vi "采水流程.vi"(11 "参数设置":cluster{"排空时间":dbl, "润洗时间":dbl, "进样超时时间":dbl}={"排空时间"=120.0, "润洗时间"=120.0, "进样超时时间"=300.0}) -> ()   [LabVIEW 2016, in "环境动力单元.lvlib"]
panel:
  in  "排空初始化":bool
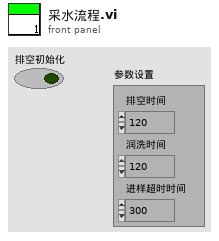
[diagram p1: front panel]
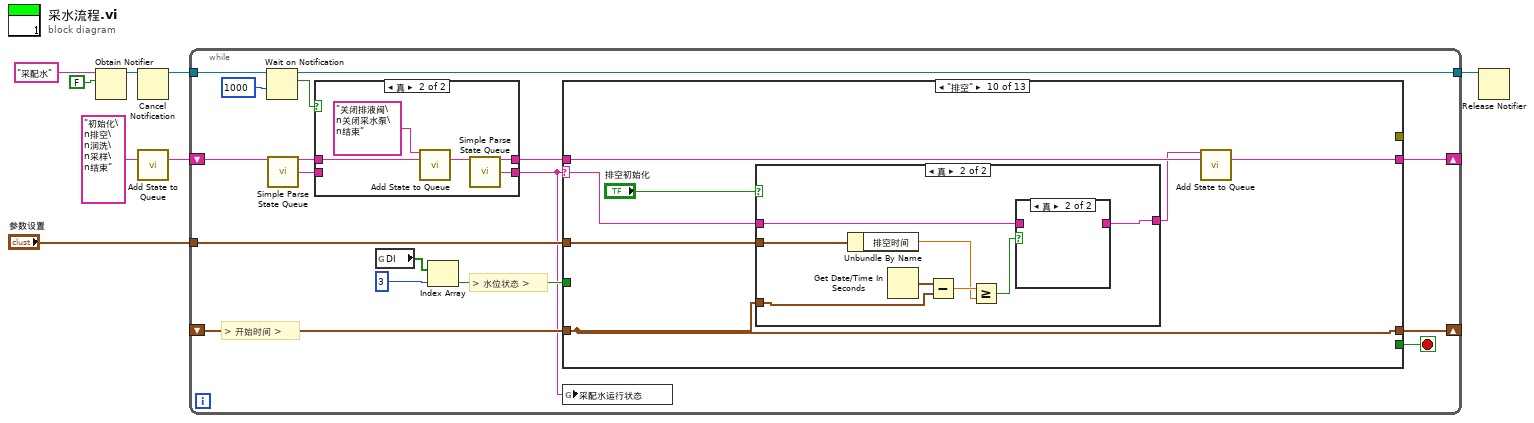
[diagram p0: block diagram]
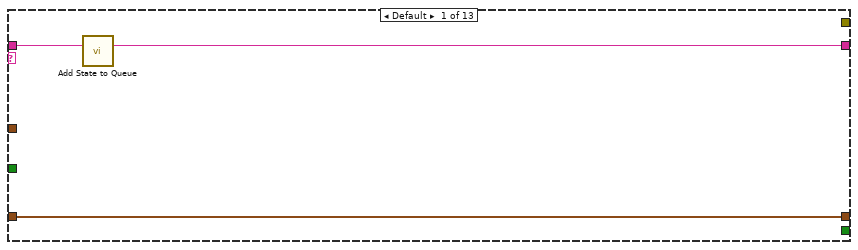
[diagram p3: hidden frame]
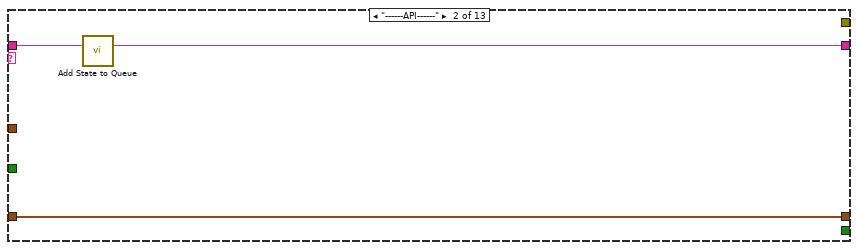
[diagram p4: hidden frame]
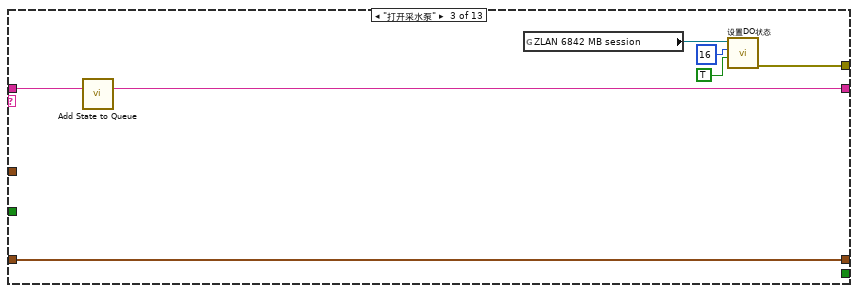
[diagram p5: hidden frame]
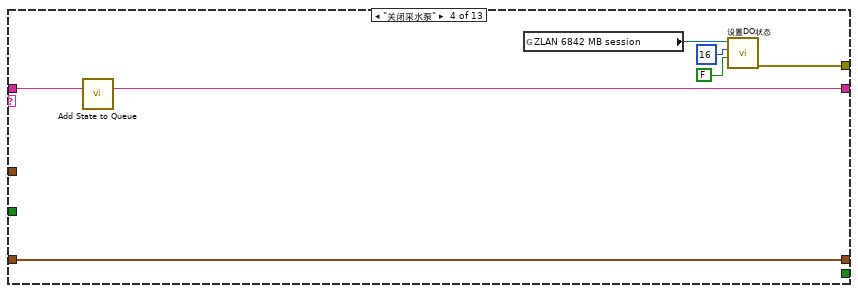
[diagram p6: hidden frame]
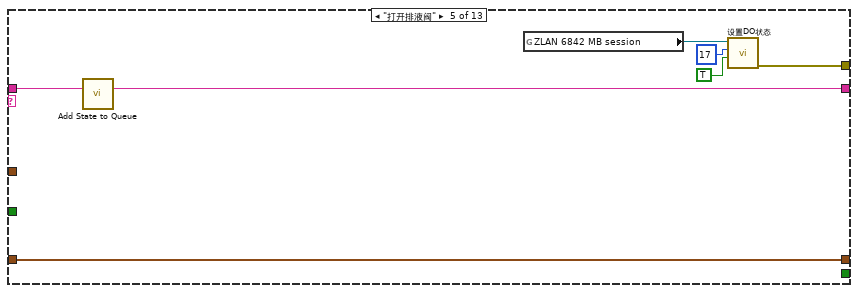
[diagram p7: hidden frame]
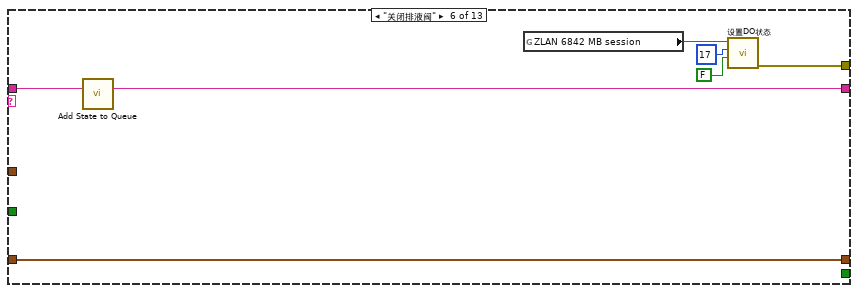
[diagram p8: hidden frame]
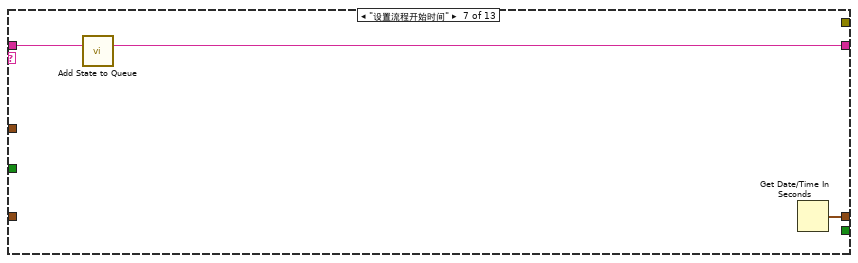
[diagram p9: hidden frame]
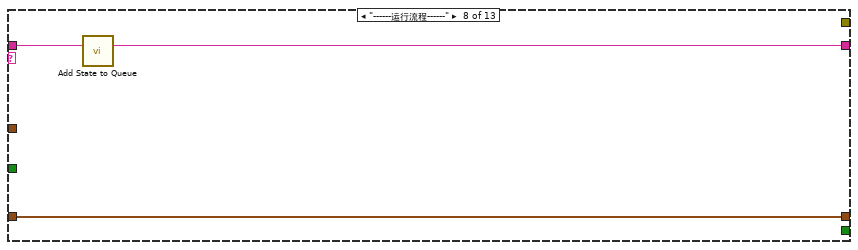
[diagram p10: hidden frame]
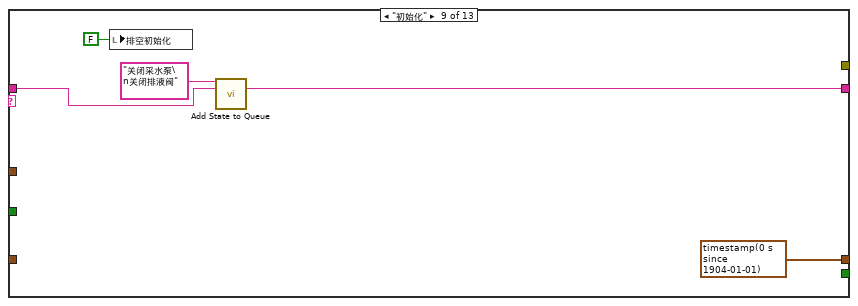
[diagram p11: hidden frame]
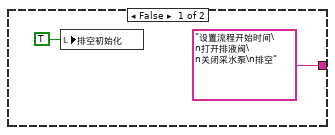
[diagram p12: hidden frame]
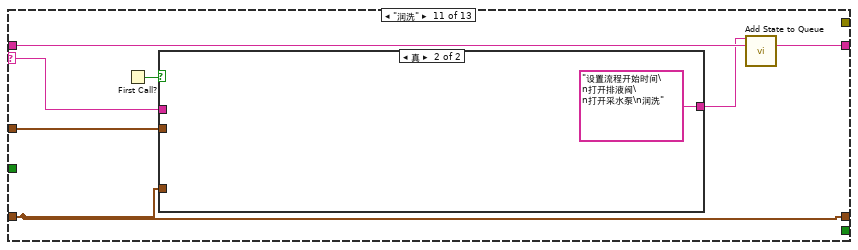
[diagram p14: hidden frame]
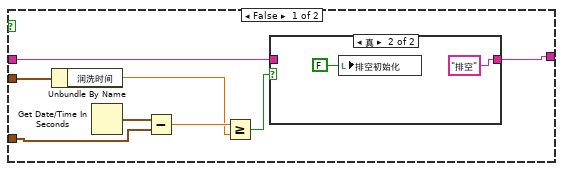
[diagram p15: hidden frame]
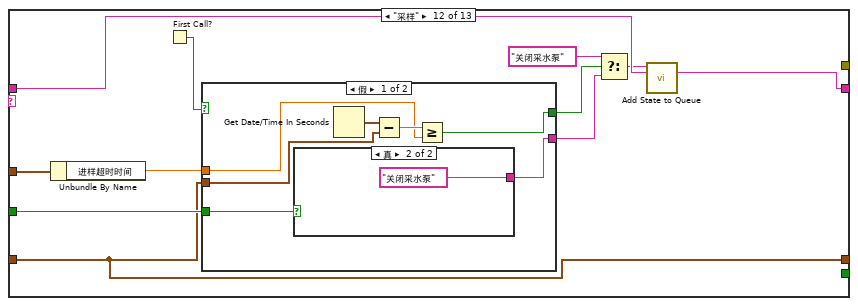
[diagram p17: hidden frame]
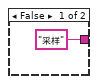
[diagram p18: hidden frame]
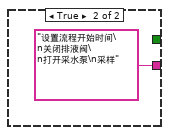
[diagram p19: hidden frame]
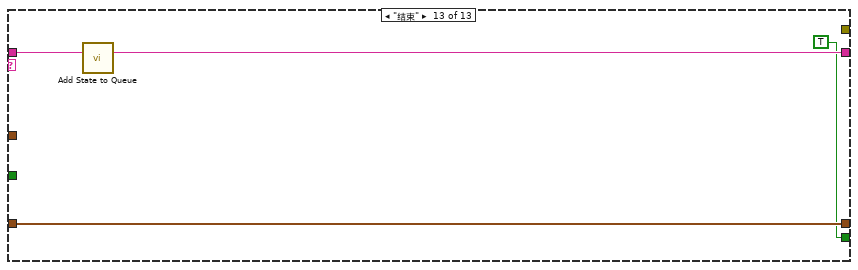
[diagram p20: hidden frame]
diagram:
  n1 = Obtain Notifier(name (unnamed)="采配水" ("名称（未命名）"), notification data type=FALSE) -> (notifier out=w3:refnum<notifier>)  [unwired: 2 in, 2 out]
  n2 = Cancel Notification(0:w3) -> (8:w2:refnum<notifier>)  [unwired: 1 in, 2 out]
  n3 = call "Add State to Queue.vi"("State(s) In (\"\")"="初始化\n排空\n润洗\n采样\n结束" ("State(s) In (\"\")")) -> ("States Out"=w7:string)  [unwired: 14 in]
  n4 = while {
    shift-right: [w24] -> _
    shift-left: w7 -> [w25]
    shift-right: [w23] -> _
    shift-left: _ -> [w22]
    tunnel: "参数设置" -> [w17]
    tunnel: w2 -> [w16]
    tunnel: [w11] -> w1
    stop <- w21 stop-if-true
    # "> 开始时间 >"
    # "> 水位状态 >"
    n5 = Wait on Notification(notifier=w16, timeout in ms (-1)=1000 ("超时毫秒(-1)")) -> (notifier out=w11:refnum<notifier>, notification=w14:bool)  [unwired: 2 in, 2 out]
    n6 = call "Simple Parse State Queue.vi"("State Queue"=w25) -> ("Remain States"=w10:string, "Next State"=w13:string)  [unwired: 13 in]
    n7 = case shown="真" w14 {
      tunnel: [w27 w29] -> w12
      tunnel: w13 -> [w27 _]
      tunnel: w10 -> [w26 w31]
      tunnel: [w26 w28] -> w9
      frame False {
      }
      frame True {
        n8 = call "Add State to Queue.vi"("State(s) In Front (\"\")"="关闭排液阀\n关闭采水泵\n结束" ("State(s) In (\"\")"), "State(s) In (\"\")"=w31) -> ("States Out"=w30:string)  [unwired: 13 in]
        n9 = call "Simple Parse State Queue.vi"("State Queue"=w30) -> ("Remain States"=w28:string, "Next State"=w29:string)  [unwired: 13 in]
      }
    }
    n10 = global read "通讯全局变量.vi" "DI"() -> (w20:bool[])
    n11 = Index Array(array=w20, index=3 ("索引")) -> (element=w18:bool)
    n12 = case shown="\"排空\"" w12 {
      selector: w12 -> [_ _ _ _ _ _ _ _ _ w81 w97 _ _]
      tunnel: w9 -> [w35 w38 w45 w52 w59 w66 w69 w72 w77 w84 w99 w125 w139]
      tunnel: [w34 w37 w44 w51 w58 w65 w68 w71 w76 w83 w102 w124 w138] -> w24
      tunnel: w18 -> [_ _ _ _ _ _ _ _ _ _ _ w123 _]
      tunnel: [_ _ w40 w47 w54 w61 _ _ _ _ _ _ _] -> _
      tunnel: [w33 w36 w39 w46 w53 w60 w67 w70 timestamp(0 s since 1904-01-01) ("seconds since 1Jan1904") w82 w100 w117 w137] -> w23
      tunnel: w22 -> [w33 w36 w39 w46 w53 w60 _ w70 _ w82 w100 w117 w137]
      tunnel: [_ _ _ _ _ _ _ _ _ _ _ _ TRUE] -> w21
      tunnel: w17 -> [_ _ _ _ _ _ _ _ _ w78 w96 w122 _]
      frame Default {
        n13 = call "Add State to Queue.vi"("State(s) In (\"\")"=w35) -> ("States Out"=w34:string)  [unwired: 14 in]
      }
      frame "------API------" {
        n14 = call "Add State to Queue.vi"("State(s) In (\"\")"=w38) -> ("States Out"=w37:string)  [unwired: 14 in]
      }
      frame "打开采水泵" {
        n15 = call "Add State to Queue.vi"("State(s) In (\"\")"=w45) -> ("States Out"=w44:string)  [unwired: 14 in]
        n16 = global read "通讯全局变量.vi" "ZLAN 6842 MB session"() -> (w41:refnum<class "MB_Master.lvclass">)
        n17 = call "设置DO状态.vi"("value"=TRUE, "address"=u16 16, "MB session in"=w41) -> ("error out"=w40:errorcluster)  [unwired: 7 in, 1 out]
      }
      frame "关闭采水泵" {
        n18 = call "Add State to Queue.vi"("State(s) In (\"\")"=w52) -> ("States Out"=w51:string)  [unwired: 14 in]
        n19 = global read "通讯全局变量.vi" "ZLAN 6842 MB session"() -> (w48:refnum<class "MB_Master.lvclass">)
        n20 = call "设置DO状态.vi"("value"=FALSE, "address"=u16 16, "MB session in"=w48) -> ("error out"=w47:errorcluster)  [unwired: 7 in, 1 out]
      }
      frame "打开排液阀" {
        n21 = call "Add State to Queue.vi"("State(s) In (\"\")"=w59) -> ("States Out"=w58:string)  [unwired: 14 in]
        n22 = global read "通讯全局变量.vi" "ZLAN 6842 MB session"() -> (w55:refnum<class "MB_Master.lvclass">)
        n23 = call "设置DO状态.vi"("value"=TRUE, "address"=u16 17, "MB session in"=w55) -> ("error out"=w54:errorcluster)  [unwired: 7 in, 1 out]
      }
      frame "关闭排液阀" {
        n24 = call "Add State to Queue.vi"("State(s) In (\"\")"=w66) -> ("States Out"=w65:string)  [unwired: 14 in]
        n25 = global read "通讯全局变量.vi" "ZLAN 6842 MB session"() -> (w62:refnum<class "MB_Master.lvclass">)
        n26 = call "设置DO状态.vi"("value"=FALSE, "address"=u16 17, "MB session in"=w62) -> ("error out"=w61:errorcluster)  [unwired: 7 in, 1 out]
      }
      frame "设置流程开始时间" {
        n27 = call "Add State to Queue.vi"("State(s) In (\"\")"=w69) -> ("States Out"=w68:string)  [unwired: 14 in]
        n28 = Get Date/Time In Seconds() -> (seconds since 1Jan1904=w67:timestamp)
      }
      frame "------运行流程------" {
        n29 = call "Add State to Queue.vi"("State(s) In (\"\")"=w72) -> ("States Out"=w71:string)  [unwired: 14 in]
      }
      frame "初始化" {
        n30 = local write "排空初始化"(FALSE ("排空初始化")) -> ()
        n31 = call "Add State to Queue.vi"("State(s) In Front (\"\")"="关闭采水泵\n关闭排液阀" ("State(s) In Front (\"\")"), "State(s) In (\"\")"=w77) -> ("States Out"=w76:string)  [unwired: 13 in]
      }
      frame "排空" {
        n32 = case shown="真" "排空初始化" {
          tunnel: ["设置流程开始时间\n打开排液阀\n关闭采水泵\n排空" ("State(s) In Front (\"\")") w90] -> w80
          tunnel: w82 -> [_ w91]
          tunnel: w81 -> [_ w89]
          tunnel: w78 -> [_ w88]
          frame False {
            n33 = local write "排空初始化"(TRUE ("排空初始化")) -> ()
          }
          frame True {
            n34 = Unbundle By Name(w88) -> ("排空时间"=w87:dbl)
            n35 = Get Date/Time In Seconds() -> (seconds since 1Jan1904=w92:timestamp)
            n36 = Subtract(x=w92, y=w91) -> (x-y=w93:dbl)
            n37 = Greater Or Equal?(x=w93, y=w87) -> (x >= y?=w94:bool)
            n38 = case shown="真" w94 {
              tunnel: [w95 _] -> w90
              tunnel: w89 -> [w95 _]
              frame False {
              }
              frame True {
              }
            }
          }
        }
        n39 = call "Add State to Queue.vi"("State(s) In Front (\"\")"=w80, "State(s) In (\"\")"=w84) -> ("States Out"=w83:string)  [unwired: 13 in]
      }
      frame "润洗" {
        n40 = First Call?() -> (First Call?: T/F=w101:bool)
        n41 = case shown="真" w101 {
          tunnel: [w106 "设置流程开始时间\n打开排液阀\n打开采水泵\n润洗" ("State(s) In Front (\"\")")] -> w98
          tunnel: w100 -> [w107 _]
          tunnel: w97 -> [w105 _]
          tunnel: w96 -> [w104 _]
          frame False {
            n42 = Unbundle By Name(w104) -> ("润洗时间"=w103:dbl)
            n43 = Get Date/Time In Seconds() -> (seconds since 1Jan1904=w108:timestamp)
            n44 = Subtract(x=w108, y=w107) -> (x-y=w109:dbl)
            n45 = Greater Or Equal?(x=w109, y=w103) -> (x >= y?=w110:bool)
            n46 = case shown="真" w110 {
              tunnel: [w111 "排空"] -> w106
              tunnel: w105 -> [w111 _]
              frame False {
              }
              frame True {
                n47 = local write "排空初始化"(FALSE ("排空初始化")) -> ()
              }
            }
          }
          frame True {
          }
        }
        n48 = call "Add State to Queue.vi"("State(s) In Front (\"\")"=w98, "State(s) In (\"\")"=w99) -> ("States Out"=w102:string)  [unwired: 13 in]
      }
      frame "采样" {
        n49 = Unbundle By Name(w122) -> ("进样超时时间"=w116:dbl)
        n50 = First Call?() -> (First Call?: T/F=w118:bool)
        n51 = case shown="假" w118 {
          tunnel: [w131 "设置流程开始时间\n关闭排液阀\n打开采水泵\n采样" ("State(s) In Front (\"\")")] -> w121
          tunnel: w123 -> [w132 _]
          tunnel: w117 -> [w128 _]
          tunnel: w116 -> [w127 _]
          tunnel: [w126 _] -> w115
          frame False {
            n52 = case shown="真" w132 {
              tunnel: ["采样" ("State(s) In Front (\"\")") "关闭采水泵" ("State(s) In Front (\"\")")] -> w131
              frame False {
              }
              frame True {
              }
            }
            n53 = Get Date/Time In Seconds() -> (seconds since 1Jan1904=w129:timestamp)
            n54 = Subtract(x=w129, y=w128) -> (x-y=w130:dbl)
            n55 = Greater Or Equal?(x=w130, y=w127) -> (x >= y?=w126:bool)
          }
          frame True {
          }
        }
        n56 = Select(t="关闭采水泵" ("State(s) In Front (\"\")"), s=w115, f=w121) -> (s? t:f=w120:string)
        n57 = call "Add State to Queue.vi"("State(s) In Front (\"\")"=w120, "State(s) In (\"\")"=w125) -> ("States Out"=w124:string)  [unwired: 13 in]
      }
      frame "结束" {
        n58 = call "Add State to Queue.vi"("State(s) In (\"\")"=w139) -> ("States Out"=w138:string)  [unwired: 14 in]
      }
    }
    n59 = global write "通讯全局变量.vi" "采配水运行状态"(w12) -> ()
  }
  n60 = Release Notifier(notifier=w1) -> ()  [unwired: 2 in, 3 out]
